vi "Calc Velocity Setpoints.vi"(8 "v scale":dbl=1.0, 9 "Iterations":i32, 10 "Angle":dbl, 11 "Path stuff":T1) -> (3 "setpoints":cluster{"left":dbl, "right":dbl})   [LabVIEW 2019]
doc: "A primitive controller that only accounts for error in angle"
uses:
  <vilib>/addons/control/pid/pid.llb/PID (DBL).vi
  <vilib>/addons/control/pid/NI_PID_pid.lvlib
panel:
  in  "i cant turn":dbl=1.0
  in  "ff":dbl=1.4
  in  "override":bool=TRUE
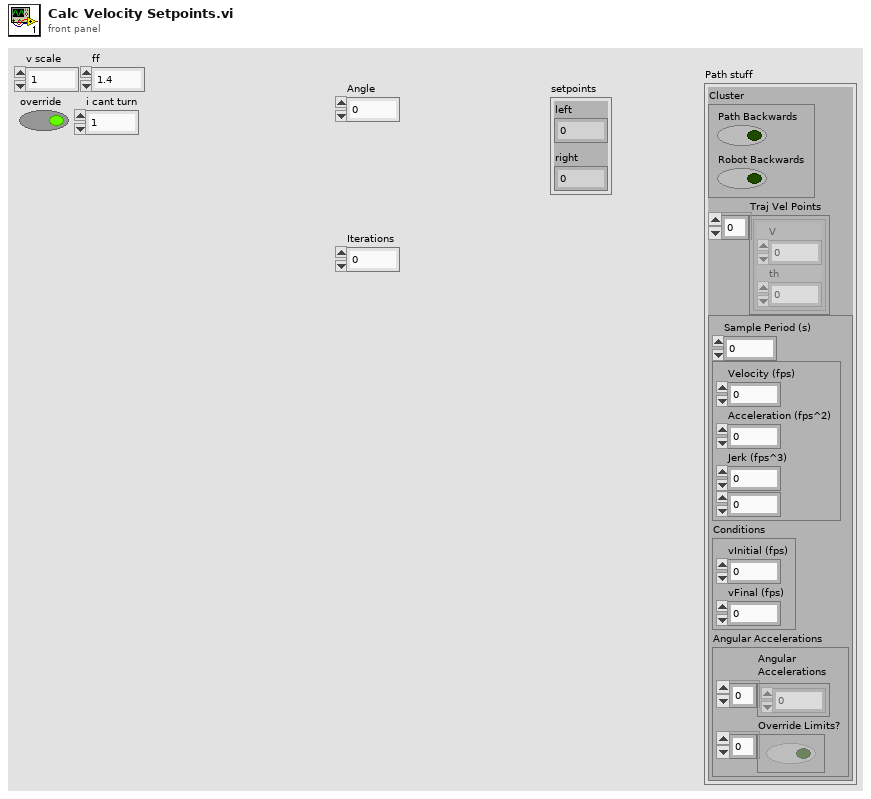
[diagram p1: front panel]
types:
  T1 = cluster{"Cluster":cluster{"Path Backwards":bool, "Robot Backwards":bool}, "Traj Vel Points":cluster{"V":dbl, "th":dbl}[], cluster{"Sample Period (s)":dbl, cluster{"Velocity (fps)":dbl, "Acceleration (fps^2)":dbl, "Jerk (fps^3)":dbl, dbl}, "Conditions":cluster{"vInitial (fps)":dbl, "vFinal (fps)":dbl}, "Angular Accelerations":cluster{"Angular \nAccelerations":dbl[], "Override Limits?":bool[]}}}
  T2 = cluster{"Path Backwards":bool, "Robot Backwards":bool}
  T3 = cluster{"proportional gain (Kc)":dbl, "integral time (Ti, min)":dbl, "derivative time (Td, min)":dbl}
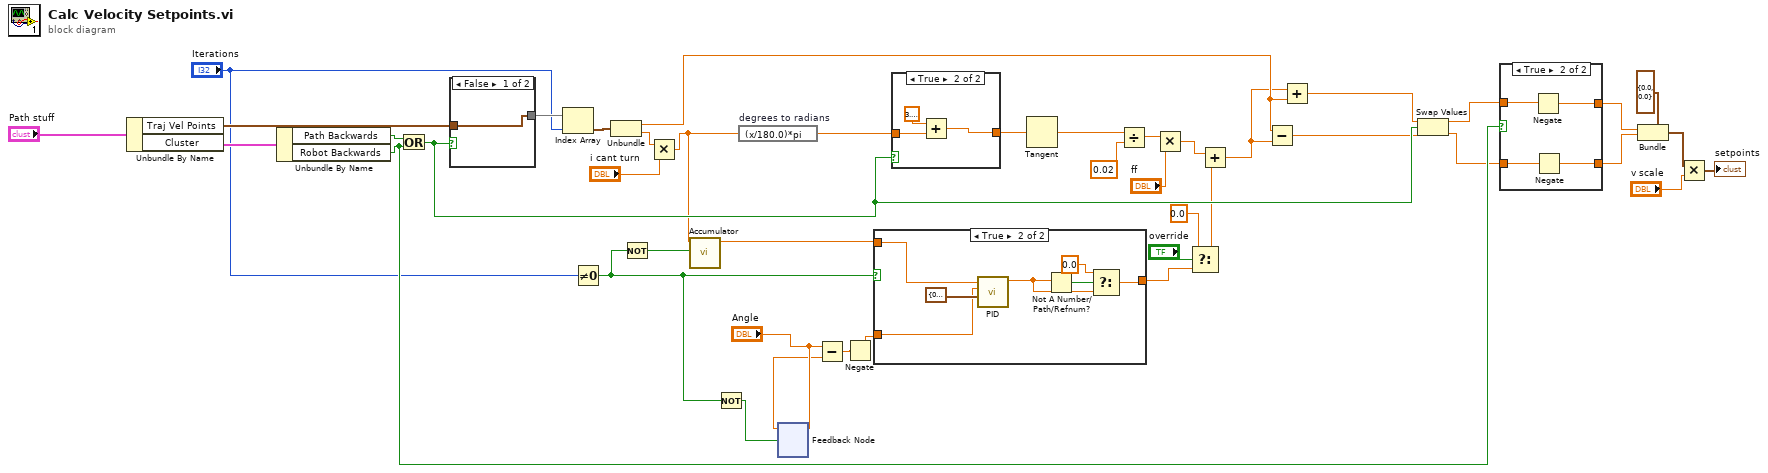
[diagram p0: block diagram]
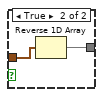
[diagram p4: hidden frame]
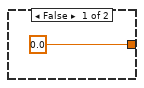
[diagram p5: hidden frame]
diagram:
  n1 = Unbundle By Name("Path stuff") -> ("Traj Vel Points"=w41:cluster{"V":dbl, "th":dbl}[], "Cluster"=w43:T2)
  n2 = Unbundle By Name(w43) -> ("Path Backwards"=w42:bool, "Robot Backwards"=w32:bool)
  n3 = Or(x=w42, y=w32) -> (x .or. y?=w33:bool)
  n4 = case shown="False" w33 {
    tunnel: w41 -> [w44 w46]
    tunnel: [w44 w45] -> w26
    frame False {
    }
    frame True {
      n5 = Reverse 1D Array(array=w46) -> (reversed array=w45:cluster{"V":dbl, "th":dbl}[])
    }
  }
  n6 = Index Array(array=w26, index="Iterations") -> (element=w40:cluster{"V":dbl, "th":dbl})
  n7 = Not Equal To 0?(x="Iterations") -> (x != 0?=w22:bool)
  n8 = Unbundle(w40) -> ("V"=w34:dbl, "th"=w11:dbl)
  n9 = Not(x=w22) -> (.not. x?=w21:bool)
  n10 = Multiply(x=w11, y="i cant turn") -> (x*y=w9:dbl)
  n11 = call "Accumulator.vi"("Reset?"=w21, "Value"=w9) -> ("Sum"=w20:dbl)  [unwired: 9 in]
  n12 = Not(x=w22) -> (.not. x?=w6:bool)
  n13 = expression code="(x/180.0)*pi" "degrees to radians"(w9) -> (w39:dbl)
  n14 = feedback-in #1("Angle", w6) -> ()
  n15 = feedback #1() -> (w4:dbl)  [unwired: 1 in]
  n16 = Subtract(x="Angle", y=w4) -> (x-y=w8:dbl)
  n17 = Negate(x=w8) -> (-x=w7:dbl)
  n18 = case shown="True" w22 {
    tunnel: w7 -> [_ w53]
    tunnel: w20 -> [_ w52]
    tunnel: [0.0 ("output") w48] -> w17
    frame False {
    }
    frame True {
      n19 = call-poly <vilib>:"PID.vi"("PID gains"=T3 {"proportional gain (Kc)"=0.08, "integral time (Ti, min)"=0.0, "derivative time (Td, min)"=0.001} ("PID gains L/S 2"), "process variable"=w53, "setpoint"=w52) -> ("output"=w50:dbl)  [unwired: 7 in, 1 out]
      n20 = Not A Number/Path/Refnum?(number/path/refnum=w50) -> (NaN/Path/Refnum?=w51:bool)
      n21 = Select(t=0.0, s=w51, f=w50) -> (s? t:f=w48:dbl)
    }
  }
  n22 = case shown="True" w33 {
    tunnel: w39 -> [w55 w58]
    tunnel: [w55 w56] -> w38
    frame False {
    }
    frame True {
      n23 = Add(x=3.141592653589793, y=w58) -> (x+y=w56:dbl)
    }
  }
  n24 = Tangent(1:w38) -> (0:w37:dbl)
  n25 = Divide(x=w37, y=0.02) -> (x/y=w35:dbl)
  n26 = Multiply(x=w35, y="ff") -> (x*y=w19:dbl)
  n27 = Select(t=0.0, s="override", f=w17) -> (s? t:f=w14:dbl)
  n28 = Add(x=w19, y=w14) -> (x+y=w18:dbl)
  n29 = Subtract(x=w34, y=w18) -> (x-y=w2:dbl)
  n30 = Add(x=w18, y=w34) -> (x+y=w3:dbl)
  n31 = Swap Values(12:w3, 13:w33, 14:w2) -> (1:w31:dbl, 3:w30:dbl)
  n32 = case shown="True" w32 {
    tunnel: w31 -> [w60 w64]
    tunnel: w30 -> [w59 w63]
    tunnel: [w60 w62] -> w28
    tunnel: [w59 w61] -> w27
    frame False {
    }
    frame True {
      n33 = Negate(x=w64) -> (-x=w62:dbl)
      n34 = Negate(x=w63) -> (-x=w61:dbl)
    }
  }
  n35 = Bundle(cluster=cluster{"left":dbl, "right":dbl} {"left"=0.0, "right"=0.0} ("setpoints"), "left"=w28, "right"=w27) -> (w24:cluster{"left":dbl, "right":dbl})
  n36 = Multiply(x=w24, y="v scale") -> (x*y=→"setpoints":cluster{"left":dbl, "right":dbl})
